vi "Configure Thermocouple [TC].vi"(8 "error in (no error)":errorcluster, 9 "ref junc type (Internal)":i32(ring)=1 items=["Internal"=1, "Fixed"=2], 10 "thermocouple type (B)":i32(ring)=1 items=["B"=1, "C"=2, "D"=3, "E"=4, "G"=5, "J"=6, "K"=7, "N"=8, "R"=9, "S"=10, "T"=11, "U"=12, "V"=13], 11 "CS++DMM in":refnum<class "CS++DMM.lvclass">) -> (0 "error out":errorcluster, 3 "CS++DMM out":refnum<class "CS++DMM.lvclass">)   [LabVIEW 2013, in "CS++DMM.lvlib" / "CS++DMM.lvclass"]
doc: "This VI configures the thermocouple type and the reference junction type of the thermocouple for DMMs that take temperature measurements using a thermocouple transducer type.\n\nThis VI affects the behavior of the instrument only if the IviDmm>Temperature Measurements>Transducer Type [TMP] property is set to IVIDMM_VAL_THERMOCOUPLE. \n\nNote:\n\n(1) This VI is part of the IviDmmThermocouple [TC] extension group."
uses:
  CS++DMM.lvclass
  Core/Classes/CS++ProcessVariables/ProcessVariable/PV.lvclass
  CS++DMM.lvclass/CS++DMM.ctl
  Core/Classes/CS++ProcessVariables/PVConnection/PVConnection.lvclass
  Core/Classes/CS++ProcessVariables/ProcessVariable/PV.lvclass/PV.ctl
  Core/Classes/CS++ProcessVariables/ProcessVariable/Write Data.vi
  Core/Classes/CS++ProcessVariables/ProcessVariable/Write Timestamp.vi
  Core/Classes/CS++ProcessVariables/ProcessVariable/Write Quality.vi
  Core/Classes/CS++ProcessVariables/ProcessVariable/Write status.vi
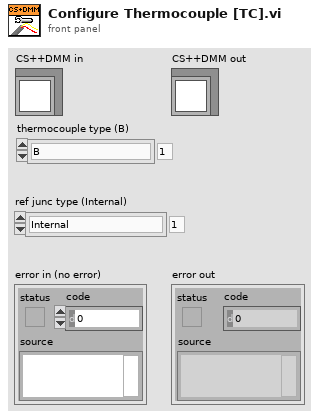
[diagram p1: front panel]
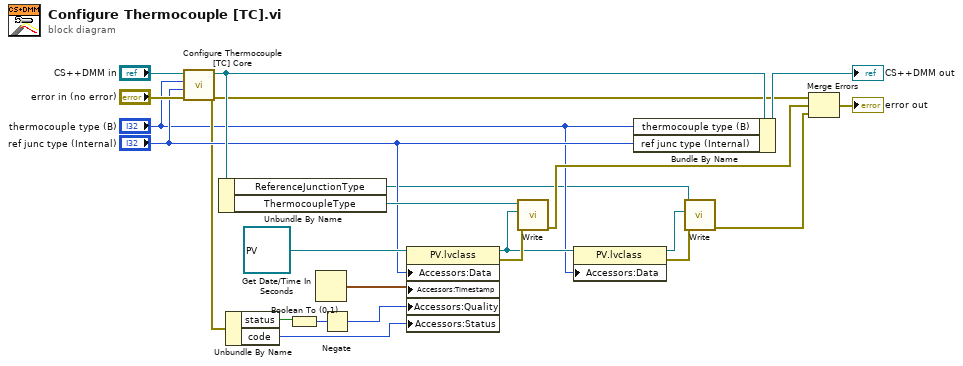
[diagram p0: block diagram]
diagram:
  n1 = call-dynamic "Configure Thermocouple [TC] Core.vi"("error in (no error)"="error in (no error)", "ref junc type (Internal)"="ref junc type (Internal)", "thermocouple type (B)"="thermocouple type (B)", "CS++DMM in"="CS++DMM in") -> ("error out"=w7:errorcluster, "CS++DMM out"=w11:refnum<class "CS++DMM.lvclass">)  [unwired: 6 in]
  n2 = Unbundle By Name(w11) -> ("ReferenceJunctionType"=w2:refnum<class "PVConnection.lvclass">, "ThermocoupleType"=w13:refnum<class "PVConnection.lvclass">)
  n3 = Unbundle By Name(w7) -> ("status"=w18:bool, "code"=w15:i32)
  n4 = Boolean To (0,1)(Boolean=w18) -> (0, 1=w17:i16)
  n5 = Get Date/Time In Seconds() -> (seconds since 1Jan1904=w14:timestamp)
  n6 = Negate(x=w17) -> (-x=w16:i16)
  n7 = property class="PV.lvclass"(reference=refnum<class "PV.lvclass"> refnum ("CS++ProcessVariables.lvlib:PV.lvclass"), "Accessors:Data"="ref junc type (Internal)", "Accessors:Timestamp"=w14, "Accessors:Quality"=w16, "Accessors:Status"=w15) -> (reference out=w5:refnum<class "PV.lvclass">, error out=w12:errorcluster)  [unwired: 1 in]
  n8 = call-dynamic "Write.vi"("error in (no error)"=w12, "PV"=w5, "PVConnection in"=w13) -> ("error out"=w6:errorcluster)  [unwired: 7 in, 1 out]
  n9 = property class="PV.lvclass"(reference=w5, "Accessors:Data"="thermocouple type (B)") -> (reference out=w8:refnum<class "PV.lvclass">, error out=w9:errorcluster)  [unwired: 1 in]
  n10 = Bundle By Name(cluster=w11, "thermocouple type (B)"="thermocouple type (B)", "ref junc type (Internal)"="ref junc type (Internal)") -> (→"CS++DMM out":refnum<class "CS++DMM.lvclass">)
  n11 = call-dynamic "Write.vi"("error in (no error)"=w9, "PV"=w8, "PVConnection in"=w2) -> ("error out"=w3:errorcluster)  [unwired: 7 in, 1 out]
  n12 = Merge Errors(w7, w6, w3) -> (→"error out":errorcluster)
